vi "计算圆心到拟合圆每个点距离.vi"(9 "Fitted Circle":T1, 11 "Img in":T2) -> (0 "铆点形状有无变异":i32, 2 "铆点数量":i32)   [LabVIEW 2014]
uses:
  <vilib>/vision/Measure.llb/Edge Options.ctl
  <vilib>/vision/Measure.llb/Edge Polarity.ctl
  <vilib>/vision/Image Controls.llb/IMAQ Image.ctl
  <vilib>/vision/NI_Vision_Development_Module.lvlib
panel:
  out "数组":i32[](array[numeric])
  out "i":i32
  out "存储当前铆点的默认位置":cluster{"X":sgl, "Y":sgl}[](array[cluster])
  out "存储铆点位置":cluster{"X":sgl, "Y":sgl}[](array[cluster])
  out "圆心到边距离 2":sgl[][](graph)
  out "输出数组 2":sgl[](array[numeric])
  in  "Options":T3={"Edge Polarity"=2, "Kernel Size"=5, "Width"=7, "Minimum Edge Strength"=20.0, "Interpolation Type"=enum."Bilinear Fixed", "Data Processing Method"=enum."Average"} {"Edge Polarity" items=["All Edges", "Rising Edges", "Falling Edges"]; "Minimum Edge Strength" format="%.2f"; "Width" step=2; "Kernel Size" step=2}
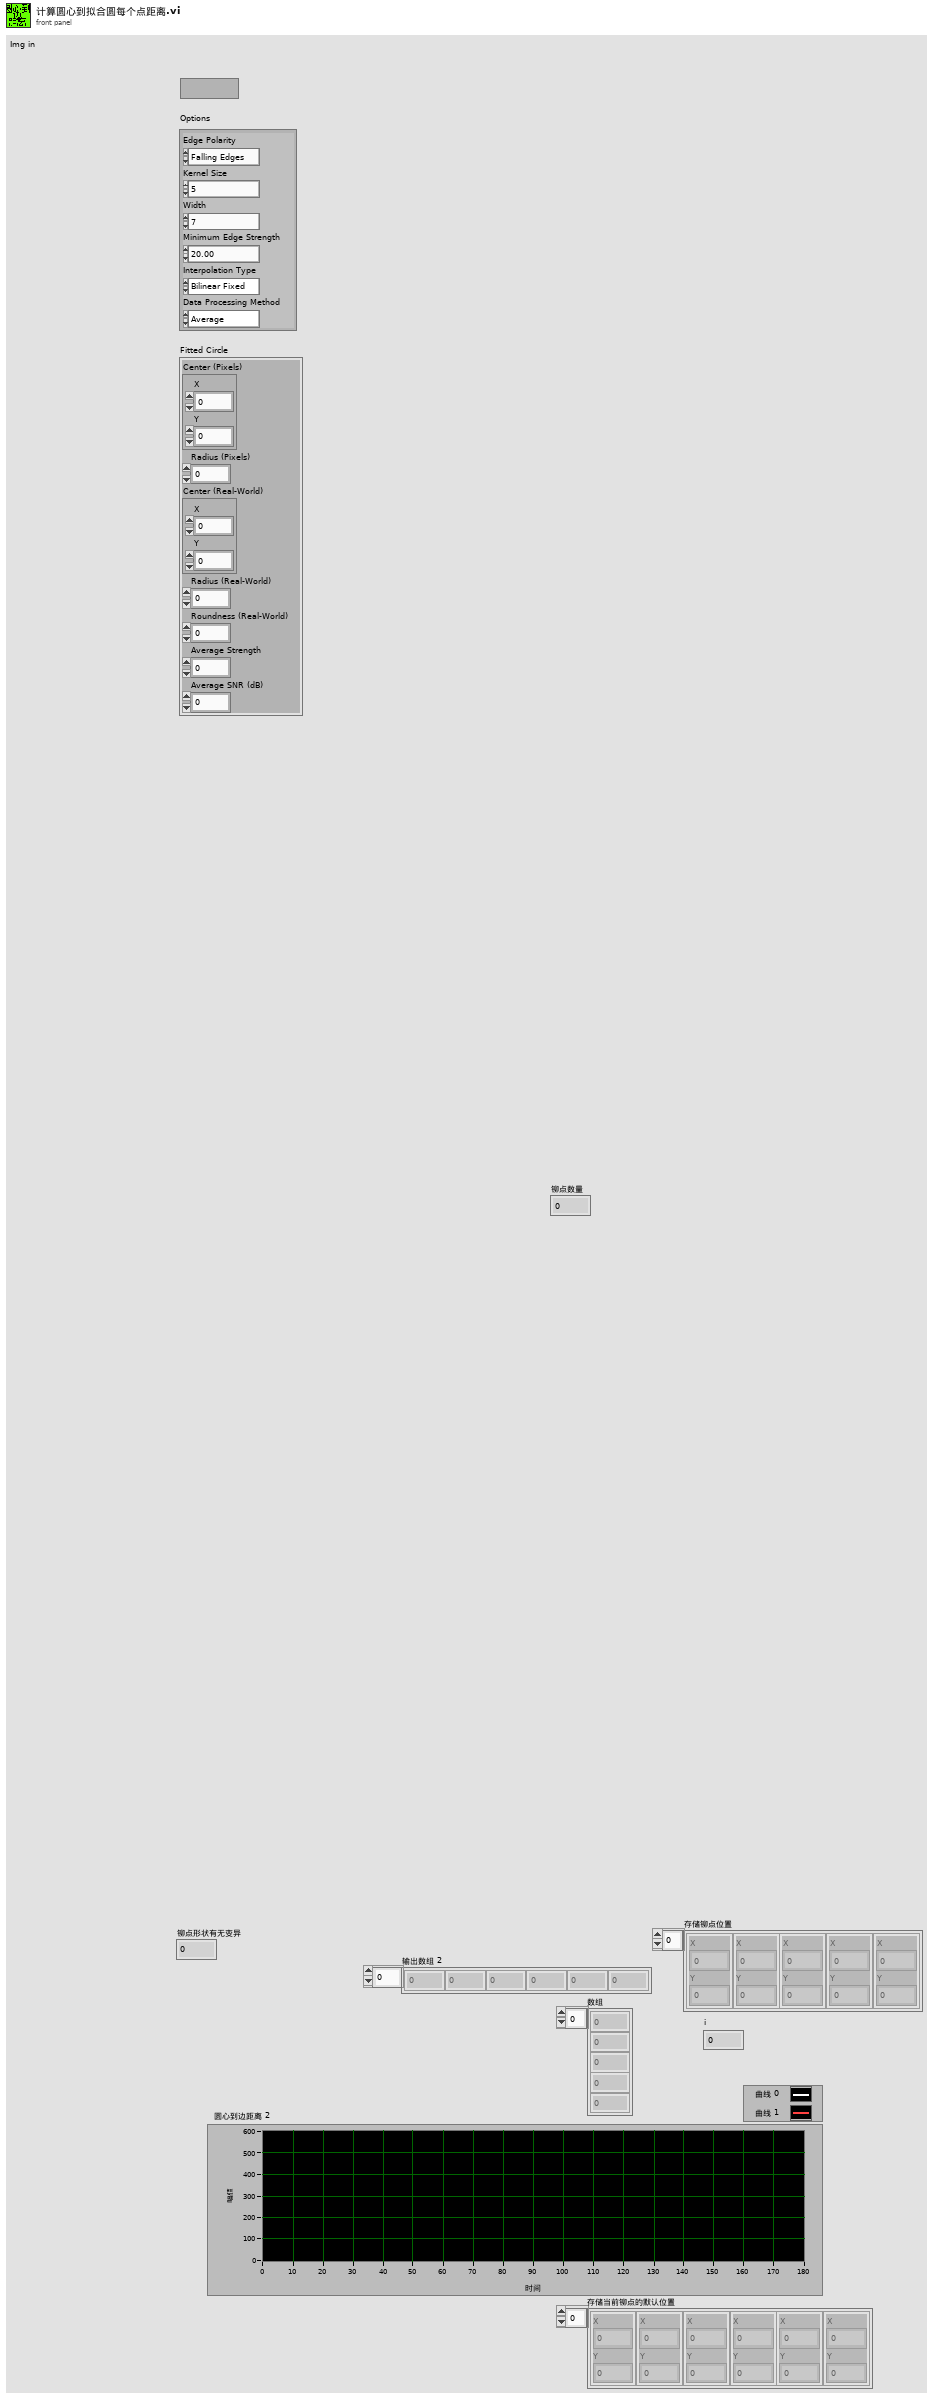
[diagram p1: front panel]
types:
  T1 = cluster{"Center (Pixels)":cluster{"X":sgl, "Y":sgl}, "Radius (Pixels)":dbl, "Center (Real-World)":cluster{"X":sgl, "Y":sgl}, "Radius (Real-World)":dbl, "Roundness (Real-World)":dbl, "Average Strength":dbl, "Average SNR (dB)":dbl}
  T2 = typedef "IMAQ Image.ctl" = refnum<image>
  T3 = typedef "Edge Options.ctl" = cluster{"Edge Polarity":T4, "Kernel Size":u32, "Width":u32, "Minimum Edge Strength":sgl, "Interpolation Type":enum32{"Zero Order", "Bilinear", "Quadratic", "Cubic", "Bilinear Fixed"}, "Data Processing Method":enum32{"Average", "Median"}}
  T4 = typedef "Edge Polarity.ctl" = u32
  T5 = enum16{"Get First Edge", "Get First + Last Edge", "Get All Edges", "Get Best Edge"}
  T6 = typedef "ROI Descriptor" = cluster{"Global Rectangle":i32[], "Contours":cluster{"ID":enum32{"External", "Internal"}, "Type":u32, "Coordinates":i32[]}[]}
  T7 = typedef "Edge New.ctl" = cluster{"Location (Pixel)":cluster{"X":sgl, "Y":sgl}, "Location (Real-World)":cluster{"X":sgl, "Y":sgl}, "Distance (Pixel)":dbl, "Distance (Real-World)":dbl, "Strength":dbl, "Noise":dbl, "Rising?":bool}
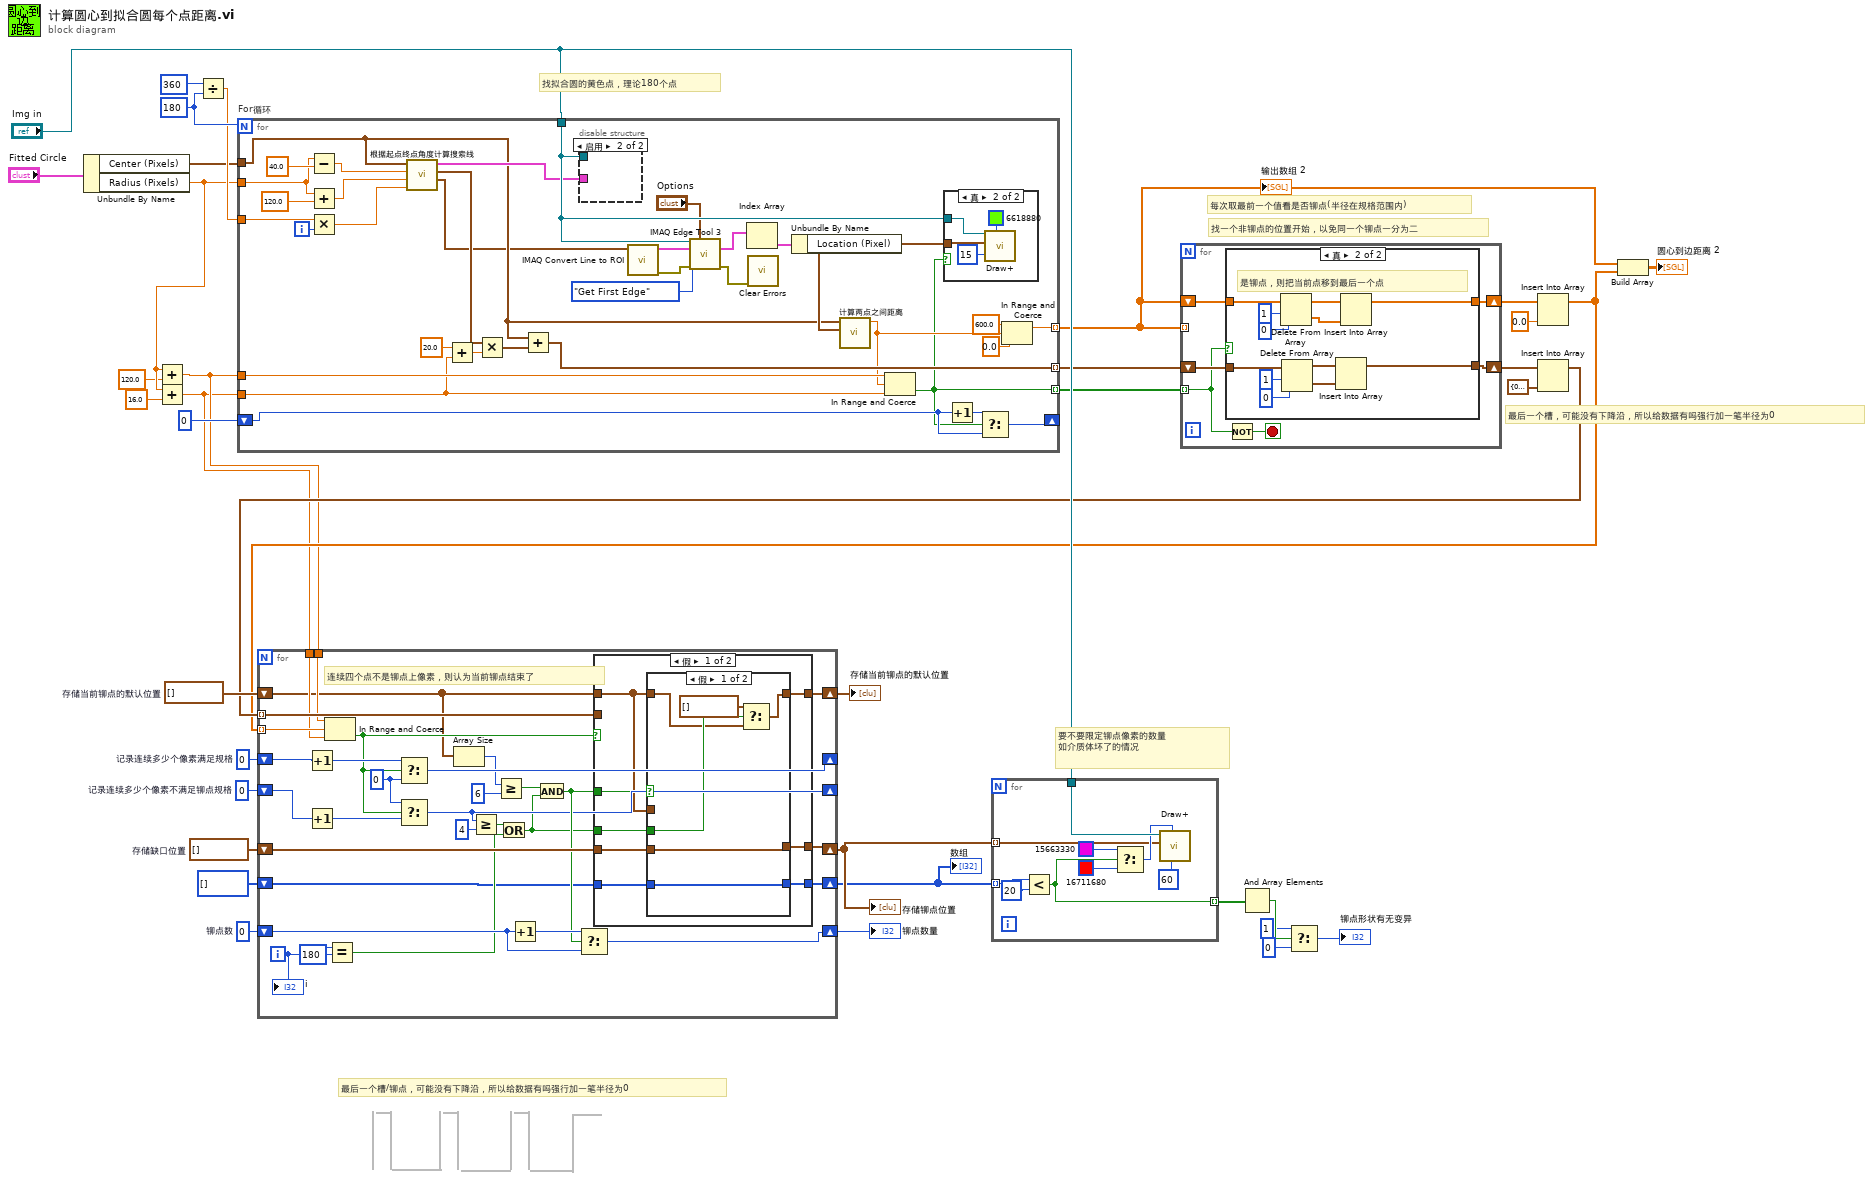
[diagram p0: block diagram]
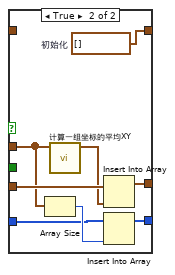
[diagram p3: hidden frame]
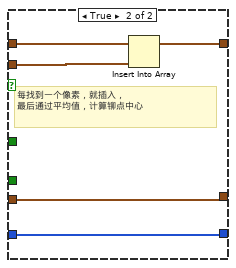
[diagram p4: hidden frame]
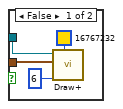
[diagram p5: hidden frame]
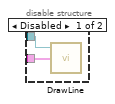
[diagram p6: hidden frame]
diagram:
  w11 = 0  # 记录连续多少个像素不满足铆点规格
  w30 = cluster{"X":sgl, "Y":sgl}[] []  # 存储缺口位置
  w31 = cluster{"X":sgl, "Y":sgl}[] []  # 存储当前铆点的默认位置
  w32 = 0  # 记录连续多少个像素满足规格
  w33 = 0  # 铆点数
  w37 = 180
  # "要不要限定铆点像素的数量\n如介质体坏了的情况"
  # "最后一个槽，可能没有下降沿，所以给数据有吗强行加一笔半径为0"
  # "每次取最前一个值看是否铆点(半径在规格范围内)"
  # "最后一个槽/铆点，可能没有下降沿，所以给数据有吗强行加一笔半径为0"
  # "找拟合圆的黄色点，理论180个点"
  # "找一个非铆点的位置开始，以免同一个铆点一分为二"
  n1 = Unbundle By Name("Fitted Circle") -> ("Center (Pixels)"=w28:cluster{"X":sgl, "Y":sgl}, "Radius (Pixels)"=w17:dbl)
  n2 = Add(x=w17, y=120.0) -> (x+y=w14:dbl)
  n3 = Add(x=w17, y=16.0) -> (x+y=w13:dbl)
  n4 = Divide(x=360, y=w37) -> (x/y=w36:dbl)
  n5 = for "For循环" {
    N: w37 -> [_]
    tunnel: w28 -> [w44]
    tunnel: "Img in" -> [w68]
    tunnel: w17 -> [w42]
    tunnel: w36 -> [w66]
    tunnel: [w59] -> w20 mode=indexing
    tunnel: [w56] -> w25 mode=indexing
    tunnel: w14 -> [w55]
    tunnel: w13 -> [w49]
    shift-right: [w53] -> _
    shift-left: 0 -> [w52]
    tunnel: [w38] -> w12 mode=indexing
    i -> [w72]
    n6 = Subtract(x=w42, y=40.0) -> (x-y=w43:dbl)
    n7 = Add(x=w42, y=120.0) -> (x+y=w40:dbl)
    n8 = Multiply(x=w66, y=w72) -> (x*y=w46:dbl)
    n9 = call "根据起点终点角度计算搜索线.vi"("角度"=w46, "外径"=w40, "内径"=w43, "Center (Pixels)"=w44) -> ("搜索线ROI"=w39:cluster{dbl, dbl, dbl, dbl}, "cos sin"=w57:cluster{dbl, dbl}, "搜索线"=w50:cluster{cluster{dbl, dbl}, cluster{dbl, dbl}})  [unwired: 5 in]
    n10 = Add(x=20.0, y=w49) -> (x+y=w47:dbl)
    n11 = Multiply(x=w57, y=w47) -> (x*y=w58:cluster{dbl, dbl})
    n12 = Add(x=w44, y=w58) -> (x+y=w56:cluster{dbl, dbl})
    n13 = disable-structure shown="启用" {
      disable-tunnel: w50 -> [w82 _]
      disable-tunnel: w68 -> [w81 _]
      frame Disabled {
        n14 = call "DrawLine.vi"("Edge Points"=w82, "img in"=w81) -> ()  [unwired: 1 in, 1 out]
      }
      frame Enabled {
      }
    }
    n15 = call "IMAQ Convert Line to ROI"("Line"=w39) -> ("error out"=w70:errorcluster, "ROI Descriptor"=w71:T6)  [unwired: 8 in]
    n16 = call "IMAQ Edge Tool 3"("Image"=w68, "Edge Options"="Options", "ROI Descriptor"=w71, "Process"=T5."Get First Edge", "error in (no error)"=w70) -> ("Edge Information"=w62:T7[], "error out"=w67:errorcluster)  [unwired: 6 in, 3 out]
    n17 = Index Array(array=w62) -> (element=w69:T7)  [unwired: 1 in]
    n18 = call <vilib>:"Clear Errors.vi"("error in (no error)"=w67) -> ()  [unwired: 5 in, 2 out]
    n19 = Unbundle By Name(w69) -> ("Location (Pixel)"=w63:cluster{"X":sgl, "Y":sgl})
    n20 = call "计算两点之间距离.vi"("Location (Pixel)"=w63, "Center (Pixels)"=w44) -> ("两点之间距离"=w51:sgl)  [unwired: 9 in]
    n21 = In Range and Coerce(upper limit=w55, x=w51, lower limit=w49) -> (In Range?=w38:bool)  [unwired: 1 out]
    n22 = case shown="真" w38 {
      tunnel: w68 -> [w75 w80]
      tunnel: w63 -> [w74 w79]
      frame False {
        n23 = call "Draw+.vi"("Width"=6, "Color"=u32 16767232, "input cluster"=w74, "Image In"=w75) -> ()  [unwired: 2 in, 1 out]
      }
      frame True {
        n24 = call "Draw+.vi"("Width"=15, "Color"=u32 6618880, "input cluster"=w79, "Image In"=w80) -> ()  [unwired: 2 in, 1 out]
      }
    }
    n25 = Increment(x=w52) -> (x+1=w54:i32)
    n26 = Select(t=w54, s=w38, f=w52) -> (s? t:f=w53:i32)
    n27 = In Range and Coerce(upper limit=sgl 600.0 ("上限"), x=w51, lower limit=sgl 0.0 ("下限")) -> (coerced(x)=w59:sgl)  [unwired: 1 out]
  }
  "输出数组 2" <- w20
  n28 = for {
    tunnel: w20 -> [_] mode=indexing
    shift-right: [w88] -> w22
    shift-left: w25 -> [w85]
    shift-right: [w87] -> w23
    shift-left: w20 -> [w84]
    tunnel: w12 -> [w83] mode=indexing
    stop <- w86 stop-if-true
    n29 = case shown="真" w83 {
      tunnel: w85 -> [w89 w102]
      tunnel: [w89 w101] -> w88
      tunnel: w84 -> [w90 w98]
      tunnel: [w90 w97] -> w87
      frame False {
      }
      frame True {
        # "是铆点，则把当前点移到最后一个点"
        n30 = Delete From Array(array=w98, length=1 ("长度"), index=0 ("索引")) -> (deleted portion=w91:sgl[], array with subset deleted=w100:sgl[])
        n31 = Delete From Array(array=w102, length=1 ("长度"), index=0 ("索引")) -> (deleted portion=w92:cluster{dbl, dbl}[], array with subset deleted=w95:cluster{dbl, dbl}[])
        n32 = Insert Into Array ("数组插入")(array=w95, new element=w92) -> (w101:cluster{dbl, dbl}[])  [unwired: 1 in]
        n33 = Insert Into Array ("数组插入")(array=w100, new element=w91) -> (w97:sgl[])  [unwired: 1 in]
      }
    }
    n34 = Not(x=w83) -> (.not. x?=w86:bool)
  }
  n35 = Insert Into Array(array=w23, new element=sgl 0.0 ("新元素/子数组")) -> (w19:sgl[])  [unwired: 1 in]
  n36 = Insert Into Array(array=w22, new element=cluster{dbl, dbl} {0.0, 0.0} ("新元素/子数组")) -> (w21:cluster{dbl, dbl}[])  [unwired: 1 in]
  n37 = for {
    tunnel: w19 -> [w122] mode=indexing
    shift-right: [w132] -> w8
    shift-left: w33 -> [w131]
    shift-right: [w117] -> _
    shift-left: w32 -> [w119]
    tunnel: w21 -> [w130] mode=indexing
    shift-right: [w129] -> w10
    shift-left: w31 -> [w109]
    shift-right: [w127] -> w9
    shift-left: w30 -> [w128]
    tunnel: w14 -> [w121]
    tunnel: w13 -> [w120]
    shift-right: [w106] -> _
    shift-left: w11 -> [w116]
    shift-right: [w105] -> w6
    shift-left: i32[] [] -> [w104]
    i -> [w123]
    w114 = 0 ("f")
    # "连续四个点不是铆点上像素，则认为当前铆点结束了"
    n38 = Increment(x=w119) -> (x+1=w118:i32)
    n39 = Increment(x=w116) -> (x+1=w115:i32)
    n40 = In Range and Coerce(upper limit=w121, x=w122, lower limit=w120) -> (In Range?=w113:bool)  [unwired: 1 out]
    n41 = Equal?(x=w123, y=180) -> (x = y?=w124:bool)
    n42 = Select(t=w118, s=w113, f=w114) -> (s? t:f=w117:i32)
    n43 = Select(t=w114, s=w113, f=w115) -> (s? t:f=w106:i32)
    n44 = Array Size(array=w109) -> (size(s)=w108:i32)
    n45 = Greater Or Equal?(x=w106, y=4) -> (x >= y?=w111:bool)
    n46 = Greater Or Equal?(x=w108, y=6) -> (x >= y?=w110:bool)
    n47 = Or(x=w111, y=w124) -> (x .or. y?=w103:bool)
    n48 = Increment(x=w131) -> (x+1=w133:i32)
    n49 = And(x=w110, y=w103) -> (x .and. y?=w126:bool)
    n50 = Select(t=w133, s=w126, f=w131) -> (s? t:f=w132:i32)
    n51 = case shown="假" w113 {
      tunnel: w109 -> [w137 w160]
      tunnel: w130 -> [_ w159]
      tunnel: [w138 w158] -> w129
      tunnel: w128 -> [w141 w157]
      tunnel: w126 -> [w139 _]
      tunnel: [w140 w157] -> w127
      tunnel: [w136 w156] -> w105
      tunnel: w104 -> [w135 w156]
      tunnel: w103 -> [w134 _]
      frame False {
        n52 = case shown="假" w139 {
          tunnel: w137 -> [_ w151]
          tunnel: w141 -> [w147 w155]
          tunnel: [w147 w153] -> w140
          tunnel: [w143 w152] -> w138
          tunnel: w137 -> [w144 _]
          tunnel: [w146 w149] -> w136
          tunnel: w135 -> [w146 w148]
          tunnel: w134 -> [w145 _]
          frame False {
            n53 = Select(t=cluster{"X":sgl, "Y":sgl}[] [], s=w145, f=w144) -> (s? t:f=w143:cluster{"X":sgl, "Y":sgl}[])
          }
          frame True {
            w152 = cluster{"X":sgl, "Y":sgl}[] []  # 初始化
            n54 = Array Size(array=w151) -> (size(s)=w150:i32)
            n55 = call "计算一组坐标的平均XY.vi"("存储当前铆点的默认位置"=w151) -> ("簇"=w154:cluster{"mean":dbl, "mean":dbl})  [unwired: 10 in]
            n56 = Insert Into Array(array=w155, new element=w154) -> (w153:cluster{"X":sgl, "Y":sgl}[])  [unwired: 1 in]
            n57 = Insert Into Array(array=w148, new element=w150) -> (w149:i32[])  [unwired: 1 in]
          }
        }
      }
      frame True {
        # "每找到一个像素，就插入，\n最后通过平均值，计算铆点中心"
        n58 = Insert Into Array(array=w160, new element=w159) -> (w158:cluster{"X":sgl, "Y":sgl}[])  [unwired: 1 in]
      }
    }
    "i" <- w123
  }
  "铆点数量" <- w8
  "存储铆点位置" <- w9
  "存储当前铆点的默认位置" <- w10
  "数组" <- w6
  n59 = for {
    tunnel: "Img in" -> [w169]
    tunnel: w9 -> [w164] mode=indexing
    tunnel: w6 -> [w163] mode=indexing
    tunnel: [w161] -> w5 mode=indexing
    n60 = Less?(x=w163, y=20) -> (x < y?=w161:bool)
    n61 = Select(t=u32 15663330 ("Color"), s=w161, f=u32 16711680 ("Color")) -> (s? t:f=w165:u32)
    n62 = call "Draw+.vi"("Width"=60, "Color"=w165, "input cluster"=w164, "Image In"=w169) -> ()  [unwired: 2 in, 1 out]
  }
  n63 = And Array Elements(Boolean array=w5) -> (logical AND=w3:bool)
  n64 = Select(t=1, s=w3, f=0) -> (s? t:f=→"铆点形状有无变异":i32)
  n65 = Build Array(w20, w19) -> (→"圆心到边距离 2":sgl[][])
